vi "Read Y_preSet.vi"(11 "reg in":refnum<class "bronkhorst_reg_2.lvclass">) -> (2 "Y_preSet":dbl, 3 "reg out":refnum<class "bronkhorst_reg_2.lvclass">)   [LabVIEW 2019, in "control.lvlib" / "bronkhorst_reg_2.lvclass"]
uses:
  bronkhorst_reg_2.lvclass
  bronkhorst_reg_2.lvclass/bronkhorst_reg_2.ctl
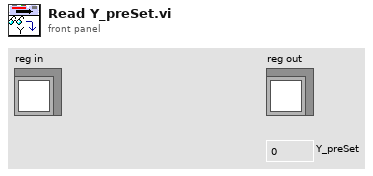
[diagram p1: front panel]
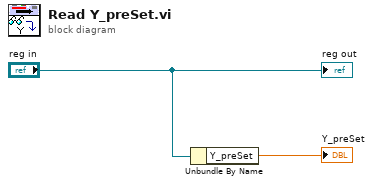
[diagram p0: block diagram]
diagram:
  n1 = Unbundle By Name("reg in") -> ("Y_preSet"=→"Y_preSet":dbl)
  "reg out" <- "reg in"
